vi "Example amier.vi"   [LabVIEW 2016]
uses:
  <vilib>/NXT/Hardware/Plugins/Tetrix DC Motor/TetrixDCMotorAddress.ctl
  <vilib>/NXT/Hardware/Plugins/Tetrix 180 deg Servo/Tetrix180ServoAddress.ctl
  <vilib>/NXT/NXTIO Xnodes/NXTIONodeSubVIs/TETRIX IO Move Servos.vi
  <vilib>/NXT/Dual Mode Library/Waits/Wait_Num.vi
  <vilib>/NXT/NXTIO Xnodes/NXTIONodeSubVIs/TETRIX IO Move DC Motors.vi
  <vilib>/NXT/NXTIO Xnodes/NXTIONodeSubVIs/TETRIX IO Stop DC Motors.vi
  <vilib>/NXT/NXTIO Xnodes/AddressXNode/NXTIOAddress.xnode
  Test.lvrbt
  <vilib>/NXT/Subs/LVHSConnector.ctl
  <vilib>/NXT/NXTIO Xnodes/NXTIOXNode/NXTIO.xnode
  <vilib>/NXT/LegoClasses/BrickReference/BrickReference.lvclass
types:
  T1 = typedef "Tetrix180ServoAddress.ctl" = i32
  T2 = cluster{"Tetrix180Servo":T1, "Tetrix180Servo":T1, "Tetrix180Servo":T1}
  T3 = typedef "LVHSConnector.ctl" = refnum<class "BrickReference.lvclass">
  T4 = typedef "TetrixDCMotorAddress.ctl" = i32
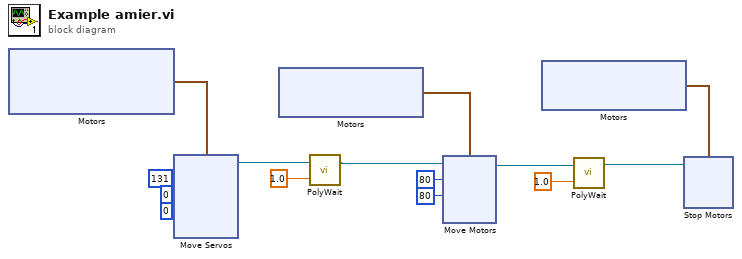
[diagram p0: block diagram]
diagram:
  n1 = xnode "Motors"() -> ("Motor"=w9:T2)
  n2 = xnode "Move Servos"("Position 3"=u8 0, "Position 2"=u8 0, "Position 1"=u8 131, "Motors"=w9) -> ("NXT/EV3"=w3:T3)  [unwired: 1 in]
  n3 = xnode "Motors"() -> ("Motor"=w14:cluster{"TetrixDCMotor":T4, "TetrixDCMotor":T4})
  n4 = call-poly <vilib>:"PolyWait.vi"("Time (1 sec)"=sgl 1.0, "NXT/EV3"=w3) -> ("NXT/EV3"=w5:T3)  [unwired: 2 in]
  n5 = xnode "Move Motors"("Power/Speed 2"=i8 80, "Power/Speed 1"=i8 80, "Motors"=w14, "NXT/EV3"=w5) -> ("NXT/EV3"=w11:T3)
  n6 = xnode "Motors"() -> ("Motor"=w2:cluster{"TetrixDCMotor":T4, "TetrixDCMotor":T4})
  n7 = call-poly <vilib>:"PolyWait.vi"("Time (1 sec)"=sgl 1.0, "NXT/EV3"=w11) -> ("NXT/EV3"=w1:T3)  [unwired: 2 in]
  n8 = xnode "Stop Motors"("Motors"=w2, "NXT/EV3"=w1) -> ()  [unwired: 1 out]
